vi "CalculateD_TypeDef.vi"(11 "Cluster In":T1) -> (3 "output cluster":T1 caption="Cluster Out")   [LabVIEW 2020]
doc: "Calculate distance from specific point to (0,0,0). Version with type def."
uses:
  Ctrl/PointCluster.ctl
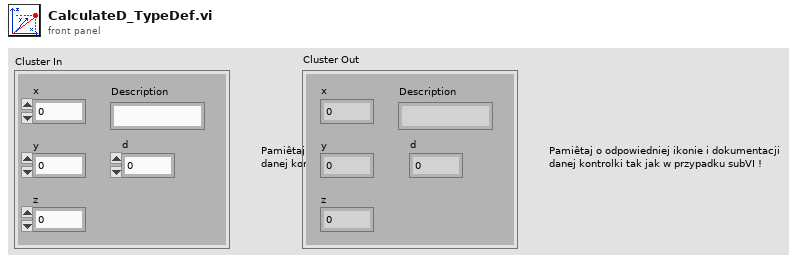
[diagram p1: front panel]
types:
  T1 = typedef "PointCluster.ctl" = cluster{"x":dbl, "y":dbl, "z ":dbl, "Description":string, "d":dbl}
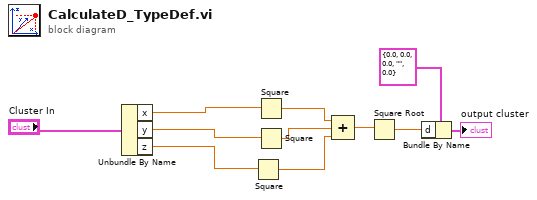
[diagram p0: block diagram]
diagram:
  n1 = Unbundle By Name("Cluster In") -> ("x"=w3:dbl, "y"=w4:dbl, "z"=w5:dbl)
  n2 = Square(x=w5) -> (x^2=w8:dbl)
  n3 = Square(x=w3) -> (x^2=w6:dbl)
  n4 = Square(x=w4) -> (x^2=w7:dbl)
  n5 = Compound Arithmetic op=ADD(w6, w7, w8) -> (w9:dbl)
  n6 = Square Root(x=w9) -> (sqrt(x)=w11:dbl)
  n7 = Bundle By Name(cluster=T1 {"x"=0.0, "y"=0.0, "z "=0.0, "Description"="", "d"=0.0} ("Cluster In 2"), "d"=w11) -> (→"output cluster":T1)
